vi "VI Tree.vi"   [LabVIEW 2023, in "Agilent B2900 Series.lvlib"]
doc: "This is the instrument driver for the Agilent B2900 Series - Keysight (Agilent) B2901A, B2902A, B2911A,B2912A, B2961A, B2962A, B2901B, B2902B, B2911B, B2912B, B2910BL, B2901BL, B2961B, B2962B. The VI Tree displays all the user-callable VIs of the instrument driver in an organized table."
uses:
  Agilent B2900 Series.lvlib
  Data/Low Level/Fetch Measurement (Multiple Points).vi
  Data/Read Measurement Result (Multiple Points).vi
  Configure/Measurement/Configure Measurement (Current).vi
  Configure/Source Output/Arbitrary Waveform/Configure Waveform (Exponential).vi
panel:
  # "(c) 2011-2025 National Instruments.  ALL RIGHTS RESERVED."
  # "SEE DIAGRAM\nFOR VI TREE."
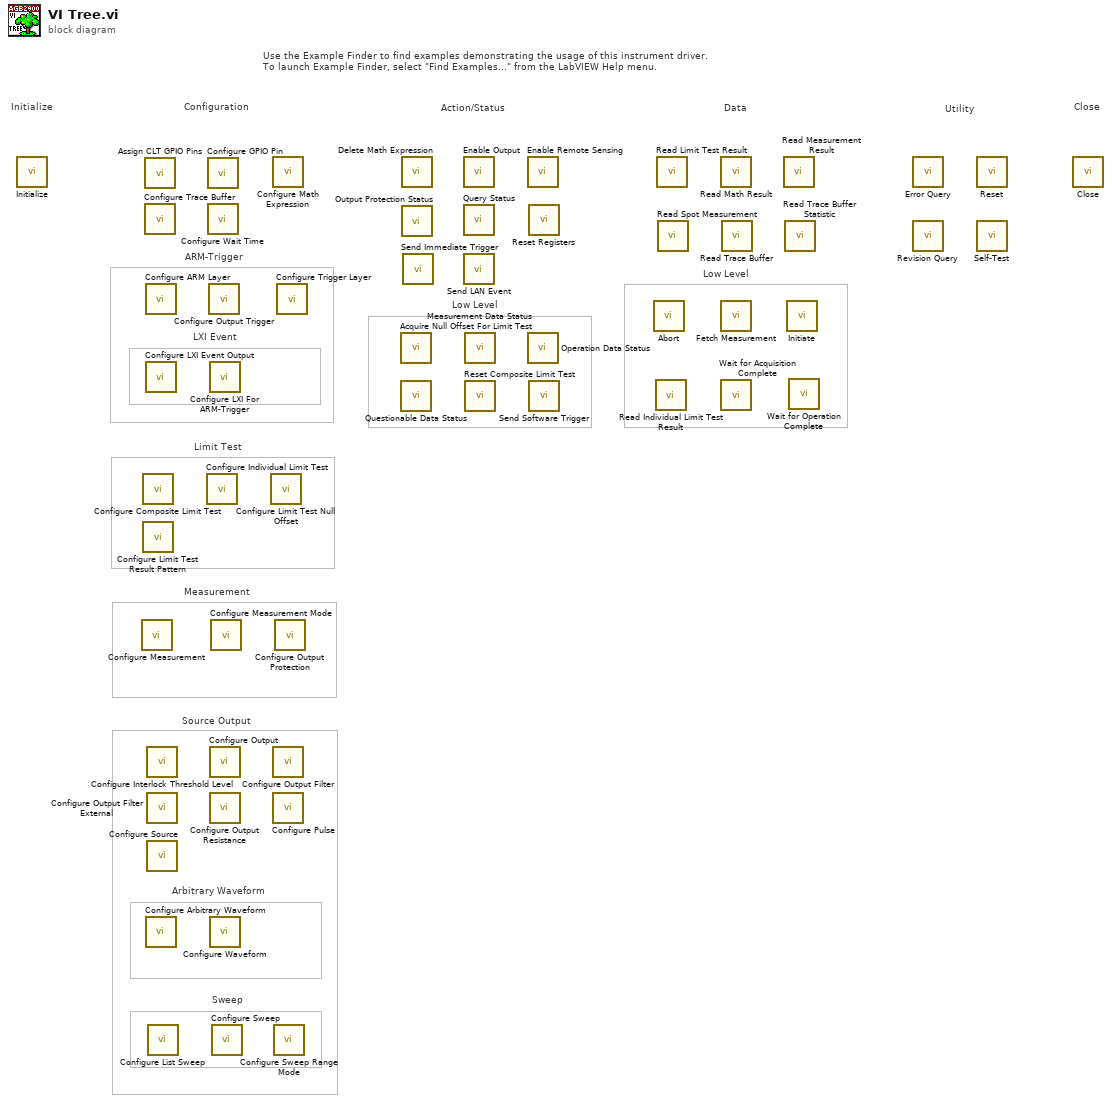
[diagram p0: block diagram]
diagram:
  # "Arbitrary Waveform"
  # "LXI Event"
  # "Low Level"
  # "Low Level"
  # "Sweep"
  # "Source Output"
  # "ARM-Trigger"
  # "Limit Test"
  # "Measurement"
  # "Use the Example Finder to find examples demonstrating the usage of this instrument driver.\nTo launch Example Finder, select \"Find Examples...\" from the LabVIEW Help menu."
  # "Configuration"
  # "Utility"
  # "Data"
  # "Action/Status"
  # "Close"
  # "Initialize"
  n1 = call "Initialize.vi"() -> ()  [unwired: 10 in, 2 out]
  n2 = call-poly "Configure Measurement.vi"() -> ()  [unwired: 18 in, 2 out]
  n3 = call "Configure Composite Limit Test.vi"() -> ()  [unwired: 14 in, 2 out]
  n4 = call "Configure Limit Test Result Pattern.vi"() -> ()  [unwired: 14 in, 2 out]
  n5 = call "Assign CLT GPIO Pins.vi"() -> ()  [unwired: 10 in, 2 out]
  n6 = call "Configure Trace Buffer.vi"() -> ()  [unwired: 10 in, 2 out]
  n7 = call "Configure ARM Layer.vi"() -> ()  [unwired: 14 in, 2 out]
  n8 = call "Configure LXI Event Output.vi"() -> ()  [unwired: 14 in, 2 out]
  n9 = call "Configure Arbitrary Waveform.vi"() -> ()  [unwired: 10 in, 2 out]
  n10 = call "Configure Interlock Threshold Level.vi"() -> ()  [unwired: 10 in, 2 out]
  n11 = call "Configure Output Filter External.vi"() -> ()  [unwired: 10 in, 2 out]
  n12 = call "Configure Source.vi"() -> ()  [unwired: 18 in, 2 out]
  n13 = call "Configure List Sweep.vi"() -> ()  [unwired: 14 in, 2 out]
  n14 = call "Configure Individual Limit Test.vi"() -> ()  [unwired: 14 in, 2 out]
  n15 = call "Configure GPIO Pin.vi"() -> ()  [unwired: 14 in, 2 out]
  n16 = call "Configure Wait Time.vi"() -> ()  [unwired: 14 in, 2 out]
  n17 = call "Configure Output Trigger.vi"() -> ()  [unwired: 14 in, 2 out]
  n18 = call "Configure LXI For ARM-Trigger.vi"() -> ()  [unwired: 14 in, 2 out]
  n19 = call "Configure Output.vi"() -> ()  [unwired: 14 in, 2 out]
  n20 = call "Configure Output Resistance.vi"() -> ()  [unwired: 14 in, 2 out]
  n21 = call-poly "Configure Waveform.vi"() -> ()  [unwired: 14 in, 2 out]
  n22 = call "Configure Measurement Mode.vi"() -> ()  [unwired: 10 in, 2 out]
  n23 = call "Configure Sweep.vi"() -> ()  [unwired: 14 in, 2 out]
  n24 = call "Configure Limit Test Null Offset.vi"() -> ()  [unwired: 10 in, 2 out]
  n25 = call "Configure Math Expression.vi"() -> ()  [unwired: 10 in, 2 out]
  n26 = call "Configure Output Filter.vi"() -> ()  [unwired: 10 in, 2 out]
  n27 = call "Configure Pulse.vi"() -> ()  [unwired: 10 in, 2 out]
  n28 = call "Configure Sweep Range Mode.vi"() -> ()  [unwired: 10 in, 2 out]
  n29 = call "Configure Output Protection.vi"() -> ()  [unwired: 10 in, 2 out]
  n30 = call "Configure Trigger Layer.vi"() -> ()  [unwired: 14 in, 2 out]
  n31 = call "Acquire Null Offset For Limit Test.vi"() -> ()  [unwired: 9 in, 3 out]
  n32 = call "Questionable Data Status.vi"() -> ()  [unwired: 9 in, 3 out]
  n33 = call "Delete Math Expression.vi"() -> ()  [unwired: 10 in, 2 out]
  n34 = call "Output Protection Status.vi"() -> ()  [unwired: 8 in, 4 out]
  n35 = call "Send Immediate Trigger.vi"() -> ()  [unwired: 10 in, 2 out]
  n36 = call "Enable Output.vi"() -> ()  [unwired: 9 in, 3 out]
  n37 = call "Query Status.vi"() -> ()  [unwired: 12 in, 4 out]
  n38 = call "Send LAN Event.vi"() -> ()  [unwired: 10 in, 2 out]
  n39 = call "Measurement Data Status.vi"() -> ()  [unwired: 9 in, 3 out]
  n40 = call "Reset Composite Limit Test.vi"() -> ()  [unwired: 10 in, 2 out]
  n41 = call "Enable Remote Sensing.vi"() -> ()  [unwired: 10 in, 2 out]
  n42 = call "Operation Data Status.vi"() -> ()  [unwired: 9 in, 3 out]
  n43 = call "Reset Registers.vi"() -> ()  [unwired: 10 in, 2 out]
  n44 = call "Send Software Trigger.vi"() -> ()  [unwired: 10 in, 2 out]
  n45 = call "Abort.vi"() -> ()  [unwired: 10 in, 2 out]
  n46 = call "Read Individual Limit Test Result.vi"() -> ()  [unwired: 9 in, 3 out]
  n47 = call "Read Limit Test Result.vi"() -> ()  [unwired: 8 in, 4 out]
  n48 = call "Read Spot Measurement.vi"() -> ()  [unwired: 9 in, 3 out]
  n49 = call "Read Math Result.vi"() -> ()  [unwired: 9 in, 3 out]
  n50 = call-poly "Fetch Measurement.vi"() -> ()  [unwired: 9 in, 3 out]
  n51 = call "Wait for Acquisition Complete.vi"() -> ()  [unwired: 10 in, 2 out]
  n52 = call "Read Trace Buffer.vi"() -> ()  [unwired: 9 in, 3 out]
  n53 = call-poly "Read Measurement Result.vi"() -> ()  [unwired: 9 in, 3 out]
  n54 = call "Read Trace Buffer Statistic.vi"() -> ()  [unwired: 9 in, 3 out]
  n55 = call "Initiate.vi"() -> ()  [unwired: 10 in, 2 out]
  n56 = call "Wait for Operation Complete.vi"() -> ()  [unwired: 10 in, 2 out]
  n57 = call "Error Query.vi"() -> ()  [unwired: 8 in, 4 out]
  n58 = call "Revision Query.vi"() -> ()  [unwired: 8 in, 4 out]
  n59 = call "Reset.vi"() -> ()  [unwired: 10 in, 2 out]
  n60 = call "Self-Test.vi"() -> ()  [unwired: 8 in, 4 out]
  n61 = call "Close.vi"() -> ()  [unwired: 11 in, 1 out]
